vi "XML_EEG_correctNumberOfDatasets.vi"(8 "error in (no error)":errorcluster, 10 "NumberOfDatasets":i32, 11 "XML_EEG_File in":refnum<class "XML_EEG_File.lvclass">) -> (0 "error out":errorcluster, 2 "DOM document out":refnum<k20>, 3 "XML_EEG_File out":refnum<class "XML_EEG_File.lvclass">)   [LabVIEW 2016, in "XML_EEG_File_Parser.lvlib" / "XML_EEG_File.lvclass"]
uses:
  XML_EEG_File.lvclass
  XML_EEG_File.lvclass/XML_EEG_File.ctl
  <vilib>/xml/NI_XML.lvlib
  <resource>/objmgr/DOMUserDefRef.rc
panel:
  # "This VI is a part of BCI Design library, http://www.ru-bci.org \nCopyright © 2020, Sotnikov Peter, All rights reserved. License: GNU GPLv3"
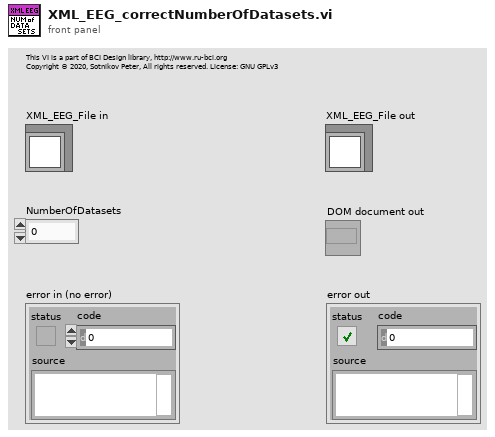
[diagram p1: front panel]
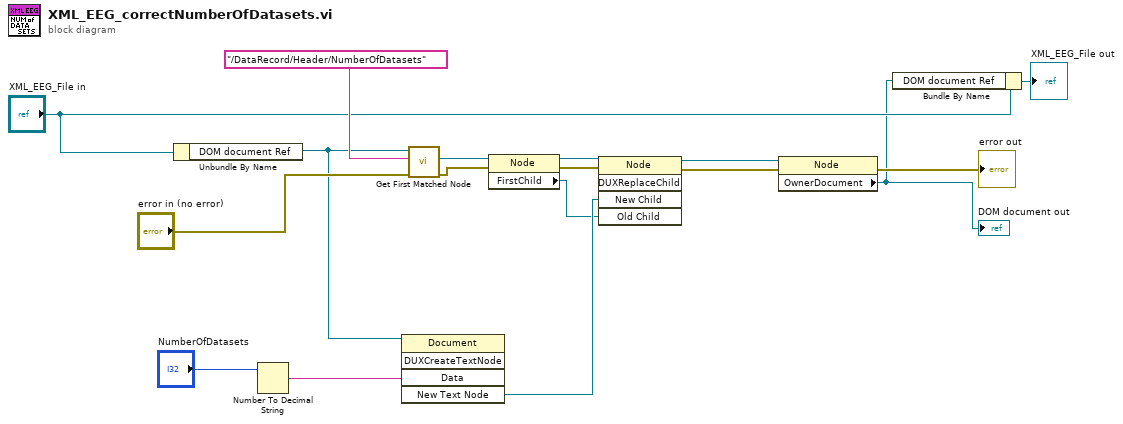
[diagram p0: block diagram]
diagram:
  n1 = Unbundle By Name("XML_EEG_File in") -> ("DOM document Ref"=w4:refnum<k20>)
  n2 = Number To Decimal String(number="NumberOfDatasets") -> (decimal integer string=w13:string)  [unwired: 1 in]
  n3 = invoke class="Document" method="DUXCreateTextNode"(reference=w4, "Data"=w13) -> ("New Text Node"=w10:refnum<k20>)  [unwired: 3 in, 4 out]
  n4 = call <vilib>:"Get First Matched Node.vi"("error in (no error)"="error in (no error)", "XPath expression"="/DataRecord/Header/NumberOfDatasets", "node in"=w4) -> ("error out"=w8:errorcluster, "node result"=w9:refnum<k20>)  [unwired: 6 in, 1 out]
  n5 = property class="Node"(reference=w9, error in=w8) -> (reference out=w7:refnum<k20>, error out=w6:errorcluster, "FirstChild"=w5:refnum<k20>)
  n6 = invoke class="Node" method="DUXReplaceChild"(reference=w7, error in=w6, "New Child"=w10, "Old Child"=w5) -> (reference out=w11:refnum<k20>, error out=w12:errorcluster)  [unwired: 1 in, 3 out]
  n7 = property class="Node"(reference=w11, error in=w12) -> (error out=→"error out":errorcluster, "OwnerDocument"=w2:refnum<k20>)  [unwired: 1 out]
  "DOM document out" <- w2
  n8 = Bundle By Name(cluster="XML_EEG_File in", "DOM document Ref"=w2) -> (→"XML_EEG_File out":refnum<class "XML_EEG_File.lvclass">)
